vi "low_pass_filter_butterworth.run.vi"(6 "Reset? (F)":bool, 7 "sampling_time (s)":dbl=2e-05, 10 "cuttoff_frequency (fc in Hz)":dbl=75.0, 11 "input":dbl format="%#_13g") -> (3 "output":dbl)   [LabVIEW 2015, in "discrete_control_systems.lvlib"]
doc: "Implements a second order low pass filter given the desired cutoff frequency (fc) and sampling time. This VI should run inline with the process acquiring the data that needs to be filtered.\n\nThe implemented low pass filer function has the following equation in the LaPlace domain, where Y(s) is the transfer function output given a U(s) intput:\n\nY(s) fc^2\n---- = ----------------------------\nU(s) s^2 + 2*0.707*fc + fc^2"
uses:
  discrete_control_systems.lvlib
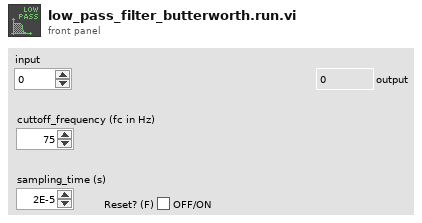
[diagram p1: front panel]
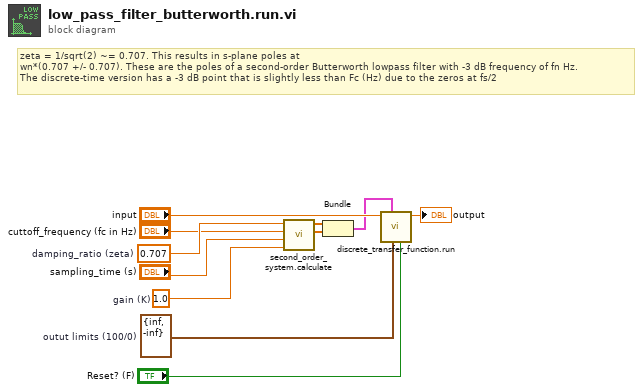
[diagram p0: block diagram]
diagram:
  w4 = cluster{"Max Limit":dbl, "Min Limit":dbl} {"Max Limit"=inf, "Min Limit"=-inf}  # outut limits (100/0)
  w6 = 1.0  # gain (K)
  w11 = 0.707  # damping_ratio (zeta)
  # "zeta = 1/sqrt(2) ~= 0.707. This results in s-plane poles at\nwn*(0.707 +/- 0.707). These are the poles of a second-order Butterworth lowpass filter with -3 dB frequency of fn Hz. \nThe discrete-time version has a -3 dB point that is slightly less than Fc (Hz) due to the zeros at fs/2"
  n1 = call "second_order_system.calculate.vi"("sampling_time (s)"=w6, "damping_ratio (zeta)"="sampling_time (s)", "natural_freq (wn in Hz)"="cuttoff_frequency (fc in Hz)", "gain (K)"=w11) -> ("a1...an"=w2:dbl[], "b0...bn"=w3:dbl[])  [unwired: 6 in]
  n2 = Bundle("b0...bn"=w3, "a1...an"=w2) -> (w1:cluster{"b0...bn":dbl[], "a1...an":dbl[]})  [unwired: 1 in]
  n3 = call "discrete_transfer_function.run.vi"("reset? (F)"="Reset? (F)", "outut limits (100/0)"=w4, "discrete_coefficients"=w1, "input"="input") -> ("output"=→"output":dbl)  [unwired: 7 in]
